vi "serialize.vi"(8 "error in":errorcluster, 10 "Waypoint In":refnum<class "Waypoint.lvclass">) -> (0 "error out":errorcluster, 2 "Flattened Waypoint":string)   [LabVIEW 2011, in "Waypoint.lvclass"]
uses:
  Waypoint.lvclass
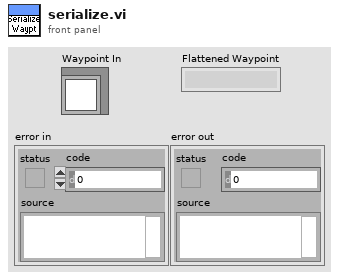
[diagram p1: front panel]
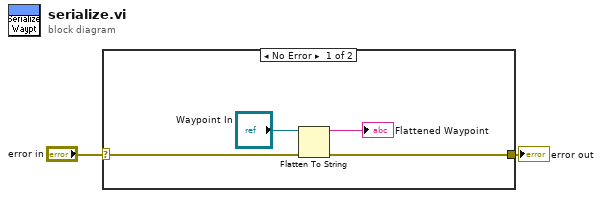
[diagram p0: block diagram]
diagram:
  n1 = case shown="No Error" "error in" {
    selector: "error in" -> [w5 w7]
    tunnel: [w6 w7] -> w2
    frame No Error {
      n2 = Flatten To String(anything="Waypoint In", error in (no error)=w5) -> (data string=→"Flattened Waypoint":string, error out=w6:errorcluster)  [unwired: 2 in, 1 out]
    }
    frame Error {
    }
  }
  "error out" <- w2
